vi "IP_生成本机局域网IP地址.vi"(8 "error in (no error)":errorcluster caption="错误输入（无错误）", 10 "第4段号码":string="188", 11 "IP地址":string caption="地址") -> (0 "error out":errorcluster caption="错误输出", 3 "本机IP地址":string)   [LabVIEW 2018]
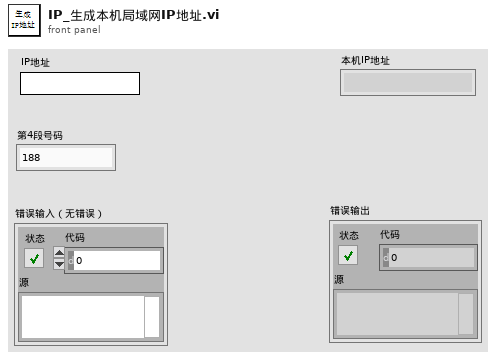
[diagram p1: front panel]
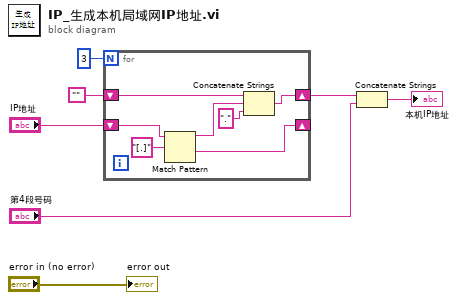
[diagram p0: block diagram]
diagram:
  n1 = for {
    N: 3 -> [_]
    shift-right: [w8] -> _
    shift-left: "IP地址" -> [w14]
    shift-right: [w10] -> w3
    shift-left: "" -> [w12]
    n2 = Match Pattern(string=w14, regular expression="[.]" ("正则表达式")) -> (before substring=w11:string, after substring=w8:string)  [unwired: 1 in, 2 out]
    n3 = Concatenate Strings(w12, w11, "." ("字符串")) -> (w10:string)
  }
  n4 = Concatenate Strings(w3, "第4段号码") -> (→"本机IP地址":string)
  "error out" <- "error in (no error)"
